vi "0716206.vi"() -> ()   [LabVIEW 2021]
panel:
  out "?":bool=TRUE
  out "Cluster 4":T1
  out "Cluster 3":T1
  out "Cluster 2":T1
  in  "input":dbl format="%#_13g"
  out "Cluster":T1
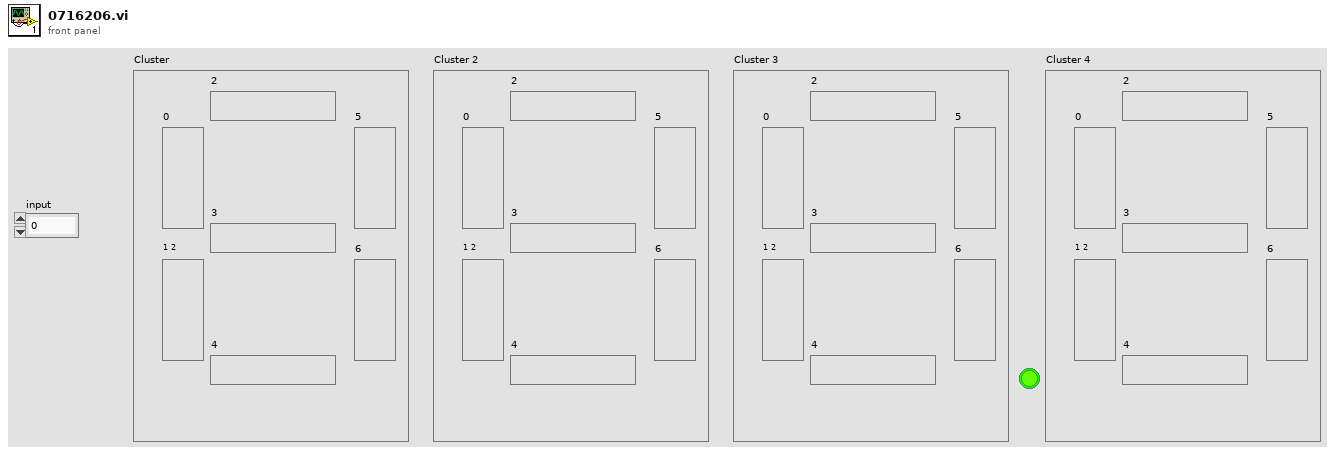
[diagram p1: front panel]
types:
  T1 = cluster{"0":bool, "1 2":bool, "2":bool, "3":bool, "4":bool, "5":bool, "6":bool, "6":bool, "6 2":bool}
  T2 = cluster{"Array 6[0]":bool, "Array 6[1]":bool, "Array 6[2]":bool, "Array 6[3]":bool, "Array 6[4]":bool, "Array 6[5]":bool, "Array 6[6]":bool, "Array 6[7]":bool, "Array 6[8]":bool}
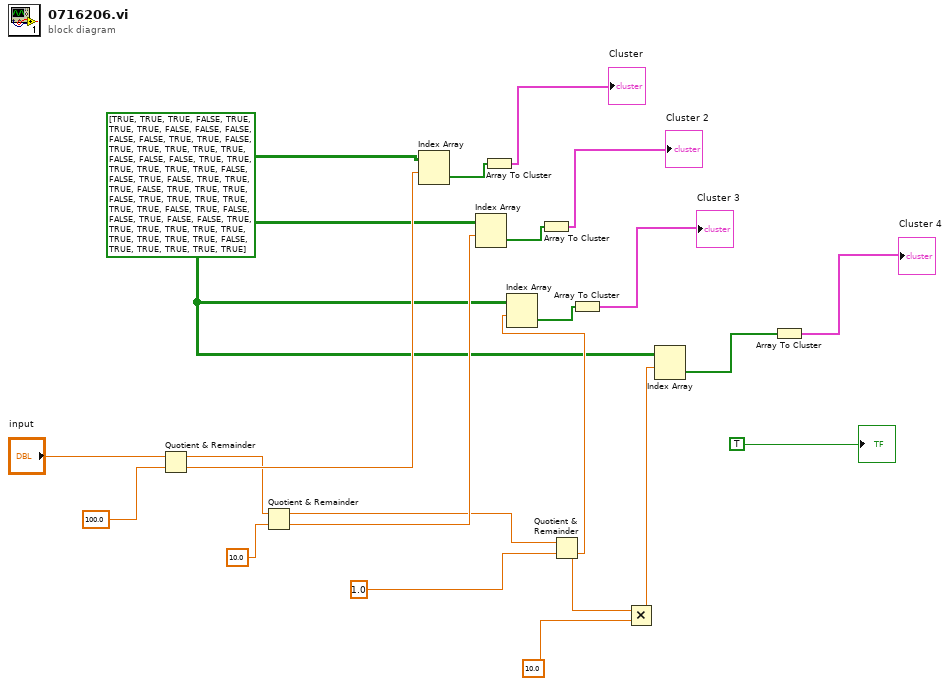
[diagram p0: block diagram]
diagram:
  w3 = bool[][] [[TRUE, TRUE, TRUE, FALSE, TRUE, TRUE, TRUE], [FALSE, FALSE, FALSE, FALSE, FALSE, TRUE, TRUE], [FALSE, TRUE, TRUE, TRUE, TRUE, TRUE, FALSE], [FALSE, FALSE, TRUE, TRUE, TRUE, TRUE, TRUE], [TRUE, FALSE, FALSE, TRUE, FALSE, TRUE, TRUE], [TRUE, FALSE, TRUE, TRUE, TRUE, FALSE, TRUE], [TRUE, TRUE, TRUE, TRUE, TRUE, FALSE, TRUE], [FALSE, FALSE, TRUE, FALSE, FALSE, TRUE, TRUE], [TRUE, TRUE, TRUE, TRUE, TRUE, TRUE, TRUE], [TRUE, FALSE, TRUE, TRUE, TRUE, TRUE, TRUE]] ("Array 6")
  n1 = Quotient & Remainder(x="input", y=100.0) -> (x-y*floor(x/y)=w12:dbl, floor(x/y)=w14:dbl)
  n2 = Quotient & Remainder(x=w12, y=10.0) -> (x-y*floor(x/y)=w9:dbl, floor(x/y)=w11:dbl)
  n3 = Index Array(array=w3, index (row)=w14) -> (element=w22:bool[])  [unwired: 1 in]
  n4 = Index Array(array=w3, index (row)=w11) -> (element=w18:bool[])  [unwired: 1 in]
  n5 = Array To Cluster(array=w22) -> (cluster=→"Cluster":T2)
  n6 = Array To Cluster(array=w18) -> (cluster=→"Cluster 2":T2)
  n7 = Quotient & Remainder(x=w9, y=1.0) -> (x-y*floor(x/y)=w6:dbl, floor(x/y)=w8:dbl)
  n8 = Index Array(array=w3, index (row)=w8) -> (element=w16:bool[])  [unwired: 1 in]
  n9 = Array To Cluster(array=w16) -> (cluster=→"Cluster 3":T2)
  n10 = Multiply(x=w6, y=10.0) -> (x*y=w2:dbl)
  n11 = Index Array(array=w3, index (row)=w2) -> (element=w5:bool[])  [unwired: 1 in]
  n12 = Array To Cluster(array=w5) -> (cluster=→"Cluster 4":T2)
  "?" <- TRUE
